vi "Write BRAND SELECTED SIM.vi"(8 "error in (no error)":errorcluster, 10 "BRAND SELECTED":enum16{"NXP", "TI", "SIMULATED"}(ring), 11 "SIMULATED in":refnum<class "SIMULATED.lvclass">) -> (0 "error out":errorcluster, 3 "SIMULATED out":refnum<class "SIMULATED.lvclass">)   [LabVIEW 2019, in "SIMULATED.lvclass"]
uses:
  SIMULATED.lvclass
  SIMULATED.lvclass/SIMULATED.ctl
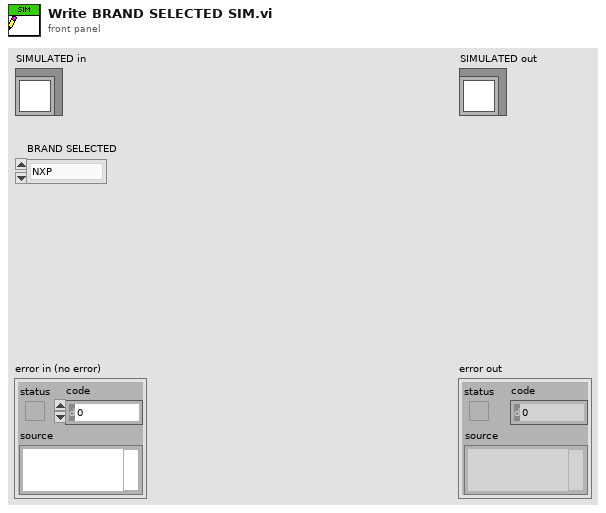
[diagram p1: front panel]
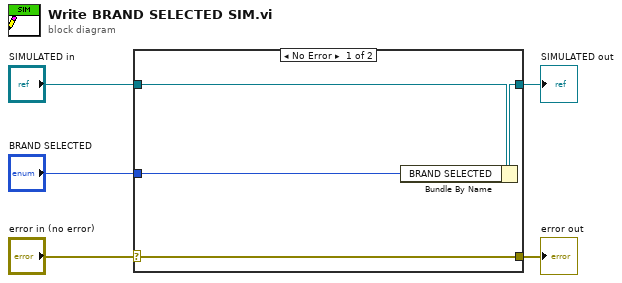
[diagram p0: block diagram]
diagram:
  n1 = case shown="No Error" "error in (no error)" {
    selector: "error in (no error)" -> [w9 w10]
    tunnel: [w9 w10] -> w4
    tunnel: [w7 w11] -> w2
    tunnel: "SIMULATED in" -> [w8 w11]
    tunnel: "BRAND SELECTED" -> [w6 _]
    frame No Error {
      n2 = Bundle By Name(cluster=w8, "BRAND SELECTED"=w6) -> (w7:refnum<class "SIMULATED.lvclass">)
    }
    frame Error {
    }
  }
  "error out" <- w4
  "SIMULATED out" <- w2
